vi "Logger-Check and Log Error.vi"(9 "error in (no error)":errorcluster, 11 "Clear?":bool) -> (10 "error out":errorcluster)   [LabVIEW 2020]
uses:
  Typedefs/Logger-Queue Data.ctl
  Typedefs/Logger-Action.ctl
  Typedefs/Logger-Level.ctl
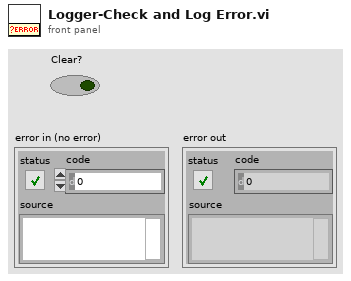
[diagram p1: front panel]
types:
  T1 = typedef "Logger-Level.ctl" = enum16{"Debug", "TCP", "Info", "Warning", "Error", "Critical"}
  T2 = typedef "Logger-Action.ctl" = enum16{"None", "Init", "Add", "Show", "Offset", "Quit"}
  T3 = typedef "Logger-Queue Data.ctl" = cluster{"Action":T2, "Level":T1, "Time":dbl, "Message":string}
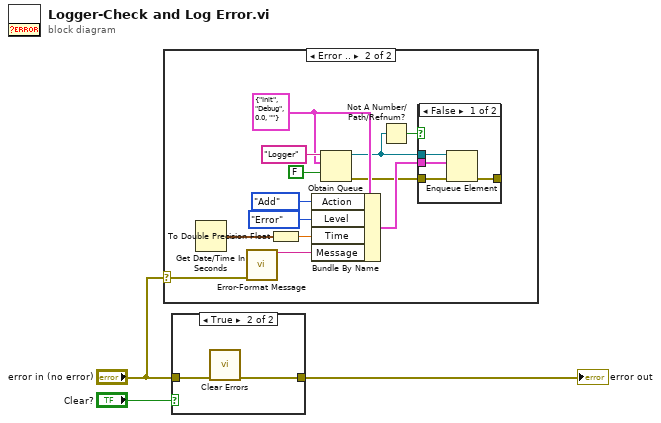
[diagram p0: block diagram]
diagram:
  n1 = case shown="Error .." "error in (no error)" {
    selector: "error in (no error)" -> [_ w4]
    frame No Error {
    }
    frame Error {
      w14 = T3 {"Action"=enum."Init", "Level"=enum."Debug", "Time"=0.0, "Message"=""} ("Trace Data")
      n2 = Get Date/Time In Seconds() -> (seconds since 1Jan1904=w10:timestamp)
      n3 = call "Error-Format Message.vi"("error in (no error)"=w4) -> ("Message"=w5:string)  [unwired: 13 in, 1 out]
      n4 = To Double Precision Float(number=w10) -> (double precision float=w11:dbl)
      n5 = Bundle By Name(cluster=w14, "Action"=Logger-Action."Add", "Level"=Logger-Level."Error", "Time"=w11, "Message"=w5) -> (w9:T3)
      n6 = Obtain Queue(name (unnamed)="Logger", element data type=w14, create if not found? (T)=FALSE) -> (queue out=w7:refnum<queue>, error out=w8:errorcluster)  [unwired: 2 in, 1 out]
      n7 = Not A Number/Path/Refnum?(number/path/refnum=w7) -> (NaN/Path/Refnum?=w6:bool)
      n8 = case shown="False" w6 {
        tunnel: w9 -> [w20 _]
        tunnel: w8 -> [w19 _]
        tunnel: w7 -> [w18 _]
        tunnel: [w17 _] -> _
        frame False {
          n9 = Enqueue Element(queue=w18, element=w20, error in (no error)=w19) -> (error out=w17:errorcluster)  [unwired: 1 in, 2 out]
        }
        frame True {
        }
      }
    }
  }
  n10 = case shown="True" "Clear?" {
    tunnel: [w21 w22] -> w2
    tunnel: "error in (no error)" -> [w21 w23]
    frame False {
    }
    frame True {
      n11 = call <vilib>:"Clear Errors.vi"("error in (no error)"=w23) -> ("error out"=w22:errorcluster)  [unwired: 5 in, 1 out]
    }
  }
  "error out" <- w2
